vi "IsWarning.vi"(2 "Numeric":i32, 3 "error string in":string) -> (0 "Error string out":string, 1 "Warning":string)   [LabVIEW 2025]
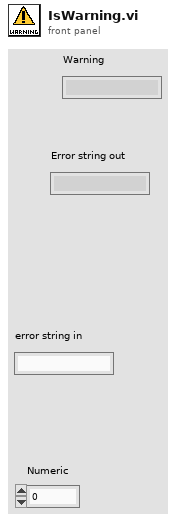
[diagram p1: front panel]
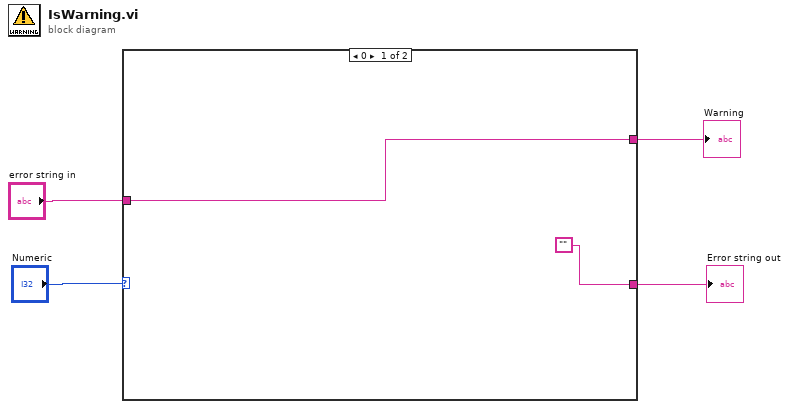
[diagram p0: block diagram]
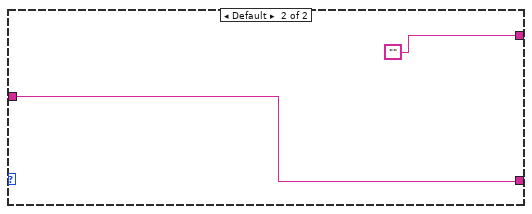
[diagram p2: hidden frame]
diagram:
  n1 = case shown="0" "Numeric" {
    tunnel: "error string in" -> [w5 w8]
    tunnel: ["" w8] -> w2
    tunnel: [w5 ""] -> w1
    frame 0 {
    }
    frame Default {
    }
  }
  "Error string out" <- w2
  "Warning" <- w1
